vi "IEEE754-to-SGL_v1.vi"(11 "Input_U8":u8[](array[numeric])) -> (3 "Output_SGL":sgl=92.92 format="%.10f")   [LabVIEW 2017]
panel:
  out "*(type *) &x":sgl format="%.10f"
  out "Exponent":i32=6
  out "Mantissa":bool[](array[boolean])=[FALSE, TRUE, TRUE, TRUE, FALSE, FALSE, TRUE, TRUE, TRUE, FALSE, TRUE, FALSE, TRUE, TRUE, TRUE, FALSE, FALSE, FALSE, FALSE, TRUE, FALSE, TRUE, FALSE]
  out "Exponent":bool[](array[boolean])=[TRUE, FALSE, FALSE, FALSE, FALSE, TRUE, FALSE, TRUE]
  out "Sign":bool
  out "Mantissa":dbl=1.4518749713897705 format="%.8f"
  out "appended array 1D":bool[](array[boolean])
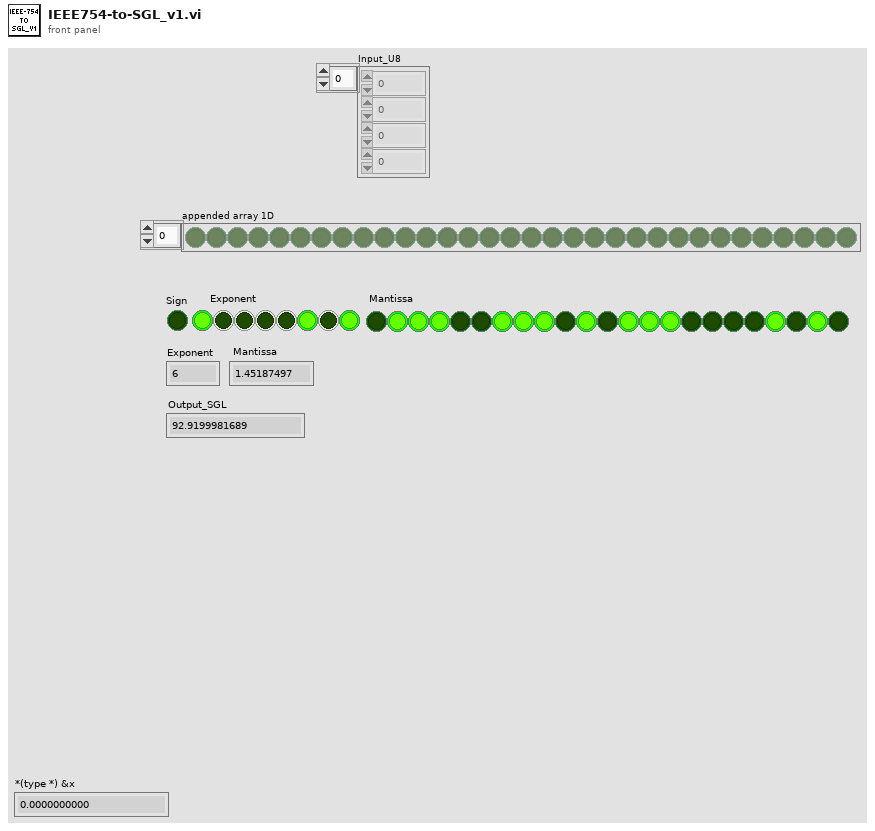
[diagram p1: front panel]
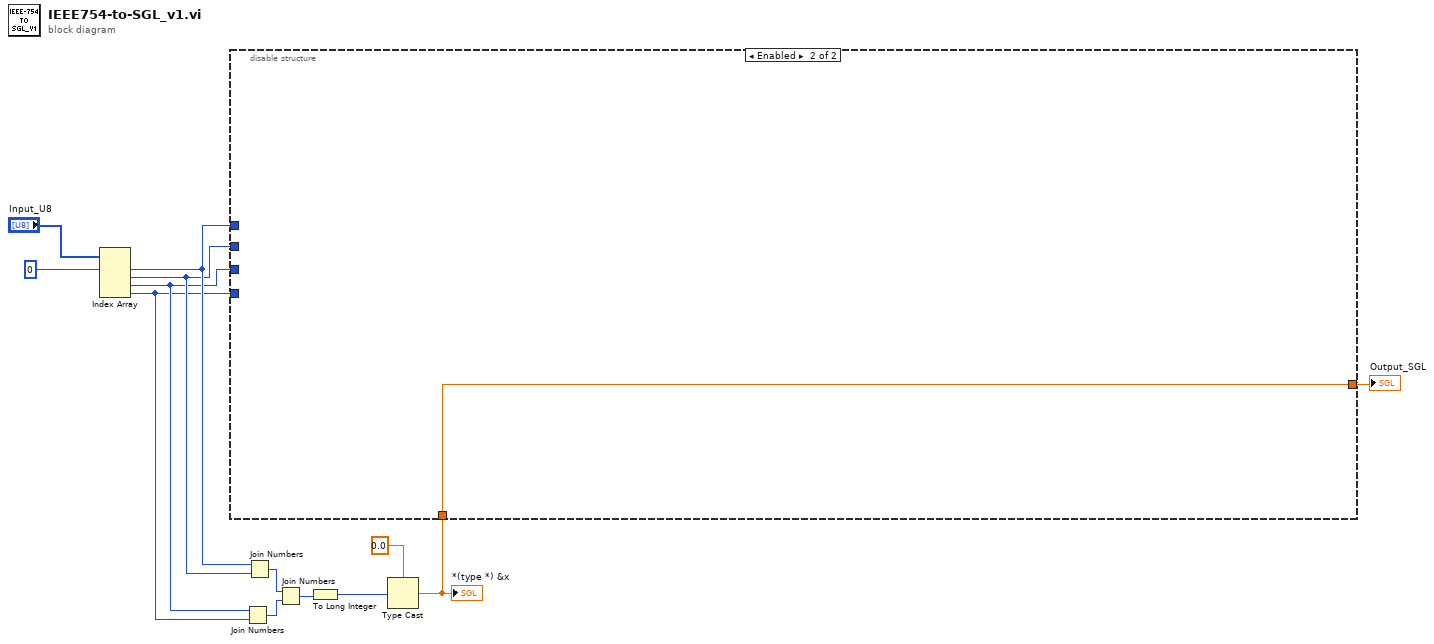
[diagram p0: block diagram]
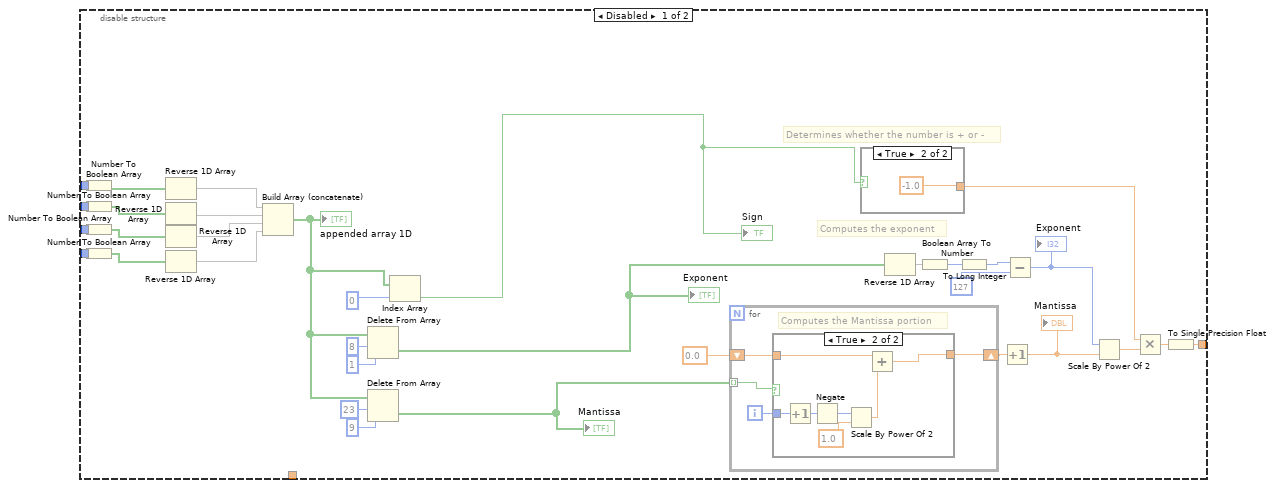
[diagram p2: hidden frame]
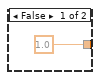
[diagram p3: hidden frame]
diagram:
  n1 = Index Array(array="Input_U8", index #1=0 ("index")) -> (element #1=w5:u8, element #2=w4:u8, element #3=w3:u8, element #4=w2:u8)  [unwired: 3 in]
  n2 = Join Numbers(hi=w3, lo=w2) -> ((hi.lo)=w8:u16)
  n3 = Join Numbers(hi=w5, lo=w4) -> ((hi.lo)=w9:u16)
  n4 = Join Numbers(hi=w9, lo=w8) -> ((hi.lo)=w7:u32)
  n5 = To Long Integer(number=w7) -> (32bit integer=w6:i32)
  n6 = Type Cast(type=sgl 0.0 ("double precision float"), x=w6) -> (*(type *) &x=w1:sgl)
  "*(type *) &x" <- w1
  n7 = disable-structure shown="Enabled" {
    disable-tunnel: [w36 w61] -> w13
    disable-tunnel: w5 -> [w17 _]
    disable-tunnel: w4 -> [w16 _]
    disable-tunnel: w3 -> [w15 _]
    disable-tunnel: w2 -> [w14 _]
    disable-tunnel: w1 -> [_ w61]
    frame Disabled {
      # "Computes the exponent"
      # "Determines whether the number is + or -"
      n8 = Number To Boolean Array(number=w17) -> (Boolean array=w26:bool[])
      n9 = Number To Boolean Array(number=w16) -> (Boolean array=w25:bool[])
      n10 = Number To Boolean Array(number=w15) -> (Boolean array=w24:bool[])
      n11 = Number To Boolean Array(number=w14) -> (Boolean array=w23:bool[])
      n12 = Reverse 1D Array(array=w26) -> (reversed array=w27:bool[])
      n13 = Reverse 1D Array(array=w25) -> (reversed array=w20:bool[])
      n14 = Reverse 1D Array(array=w24) -> (reversed array=w21:bool[])
      n15 = Reverse 1D Array(array=w23) -> (reversed array=w22:bool[])
      n16 = Build Array (concatenate)(w27, w20, w21, w22) -> (w30:bool[])
      "appended array 1D" <- w30
      n17 = Delete From Array(array=w30, length=8, index=1) -> (deleted portion=w31:bool[])  [unwired: 1 out]
      "Exponent" <- w31
      n18 = Delete From Array(array=w30, length=23, index=9) -> (deleted portion=w19:bool[])  [unwired: 1 out]
      "Mantissa" <- w19
      n19 = Index Array(array=w30, index=0) -> (element=w28:bool)
      "Sign" <- w28
      n20 = for {
        tunnel: w19 -> [w52] mode=indexing
        shift-right: [w49] -> w18
        shift-left: 0.0 -> [w50]
        i -> [w51]
        # "Computes the Mantissa portion"
        n21 = case shown="True" w52 {
          tunnel: w51 -> [_ w60]
          tunnel: w50 -> [w53 w56]
          tunnel: [w53 w54] -> w49
          frame False {
          }
          frame True {
            n22 = Increment(x=w60) -> (x+1=w59:i32)
            n23 = Negate(x=w59) -> (-x=w58:i32)
            n24 = Scale By Power Of 2(n=w58, x=1.0) -> (x*2^n=w55:dbl)
            n25 = Add(x=w56, y=w55) -> (x+y=w54:dbl)
          }
        }
      }
      n26 = case shown="True" w28 {
        tunnel: [1.0 -1.0] -> w40
        frame False {
        }
        frame True {
        }
      }
      n27 = Reverse 1D Array(array=w31) -> (reversed array=w42:bool[])
      n28 = Boolean Array To Number(Boolean array=w42) -> (number=w38:u32)
      n29 = To Long Integer(number=w38) -> (32bit integer=w37:i32)
      n30 = Increment(x=w18) -> (x+1=w44:dbl)
      "Mantissa" <- w44
      n31 = Subtract(x=w37, y=127) -> (x-y=w39:i32)
      "Exponent" <- w39
      n32 = Scale By Power Of 2(n=w39, x=w44) -> (x*2^n=w43:dbl)
      n33 = Multiply(x=w40, y=w43) -> (x*y=w41:dbl)
      n34 = To Single Precision Float(number=w41) -> (single precision float=w36:sgl)
    }
    frame Enabled {
    }
  }
  "Output_SGL" <- w13
